vi "simple_phase.vi"(11 "DOA":dbl) -> (3 "simple phase":dbl[](array[numeric]))   [LabVIEW 2021]
uses:
  <vilib>/Analysis/coordinate.llb/Angle Range (Degree).ctl
  <vilib>/Analysis/coordinate.llb/Angle Units.ctl
  <vilib>/Analysis/1siggen.llb/Ramp Pattern by Delta.vi
  <vilib>/Analysis/NI_AALBase.lvlib
  <vilib>/Analysis/NI_AAL_Angle.lvlib
  <vilib>/Analysis/coordinate.llb/Wrap Angle (array).vi
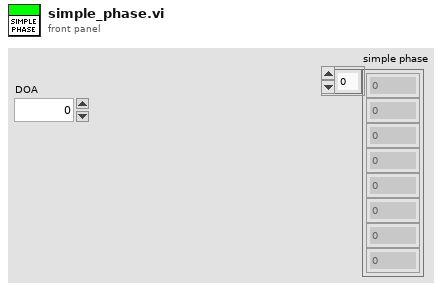
[diagram p1: front panel]
types:
  T1 = typedef "NI_AAL_Angle.lvlib/Angle Units.ctl" = i32
  T2 = typedef "NI_AAL_Angle.lvlib/Angle Range (Degree).ctl" = u16
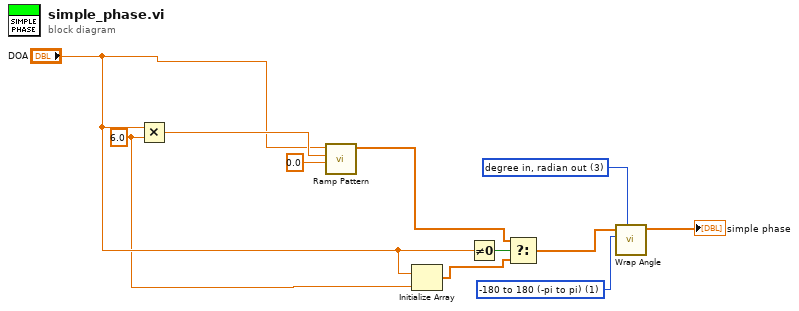
[diagram p0: block diagram]
diagram:
  w8 = T1 3 items=["radian in, radian out", "radian in, degree out", "degree in, degree out", "degree in, radian out"] ("angle units")
  w9 = T2 1 items=["none", "-180 to 180 (-pi to pi)", "0 to 360 (0 to 2pi)"] ("angle range")
  w1 = 6.0 ("y")
  n1 = Multiply(x="DOA", y=w1) -> (x*y=w10:dbl)
  n2 = call-poly <vilib>:"Ramp Pattern.vi"("start"=0.0, "end"=w10, "delta"="DOA") -> ("Ramp Pattern"=w5:dbl[])  [unwired: 6 in, 2 out]
  n3 = Initialize Array("DOA", w1) -> (w3:dbl[])
  n4 = Not Equal To 0?(x="DOA") -> (x != 0?=w6:bool)
  n5 = Select(t=w5, s=w6, f=w3) -> (s? t:f=w4:dbl[])
  n6 = call-poly <vilib>:"Wrap Angle.vi"("angle units"=w8, "angle range"=w9, "Angle In"=w4) -> ("Angle Out"=→"simple phase":dbl[])  [unwired: 7 in, 1 out]
